vi "Main.vi"() -> ()   [LabVIEW 2021]
doc: "The myRIO Project template acquires acceleration data from the onboard accelerometer and displays the changes of acceleration values in a waveform chart."
panel:
  out "PLACEHOLDER\nLED control":dbl format="%#_13g"
  in  "PLACEHOLDER\nSfc Temp":dbl=150.0 format="%#_13g"
  out "Warmer\nON":bool
  out "HOT\nSurface":bool
  out "Surface Danger Level":string
  in  "Set-Temp-Slider":dbl(slide) scale=80.0..180.0
  out "Temp-Chart":T1(graph)
  in  "stop":bool
  # "Nice Warm Coffee"
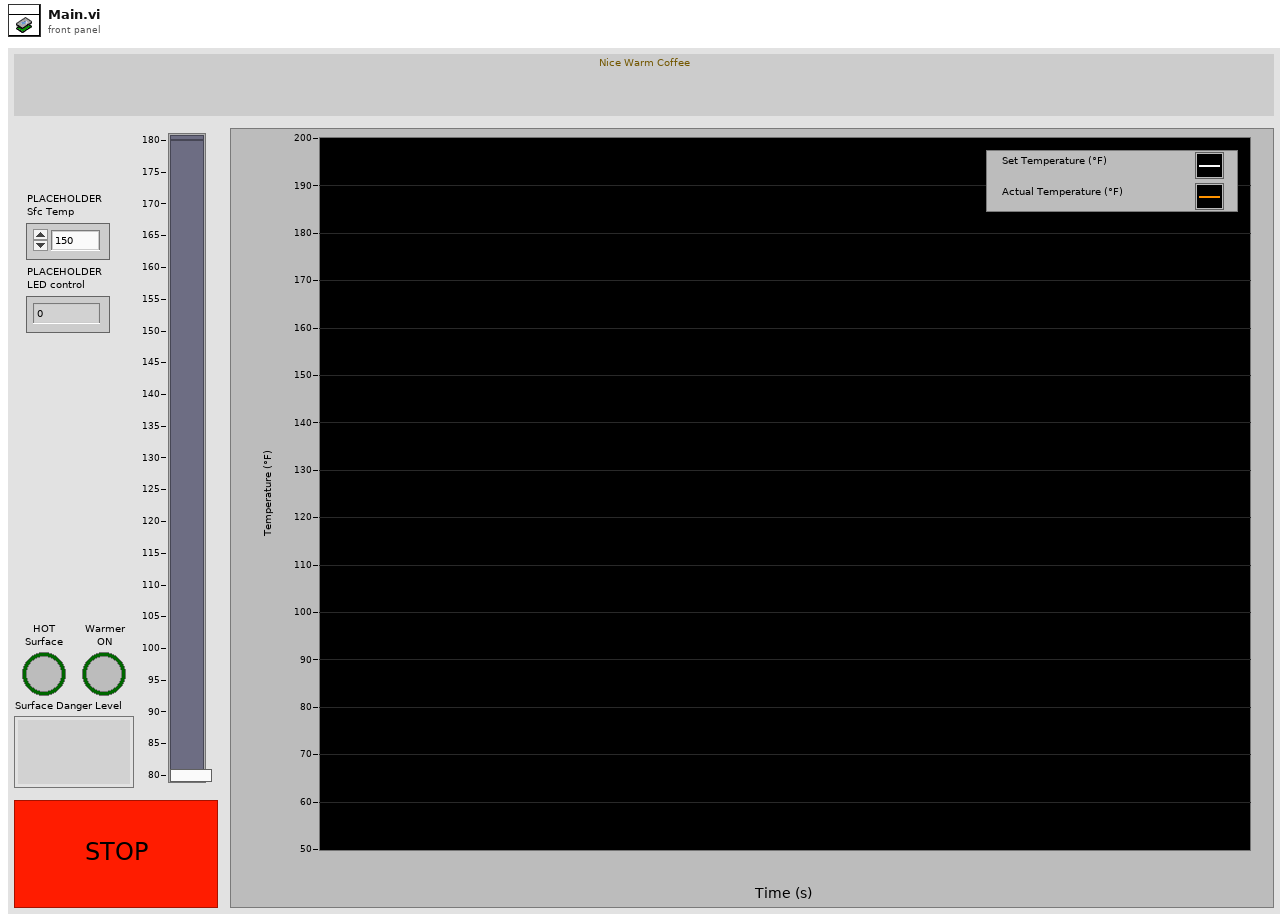
[diagram p1: front panel]
types:
  T1 = cluster{"[0]":dbl, "[1]":dbl, "[2]":dbl, "[3]":dbl, "[4]":dbl, "[5]":dbl, "[6]":dbl, "[7]":dbl, "[8]":dbl}
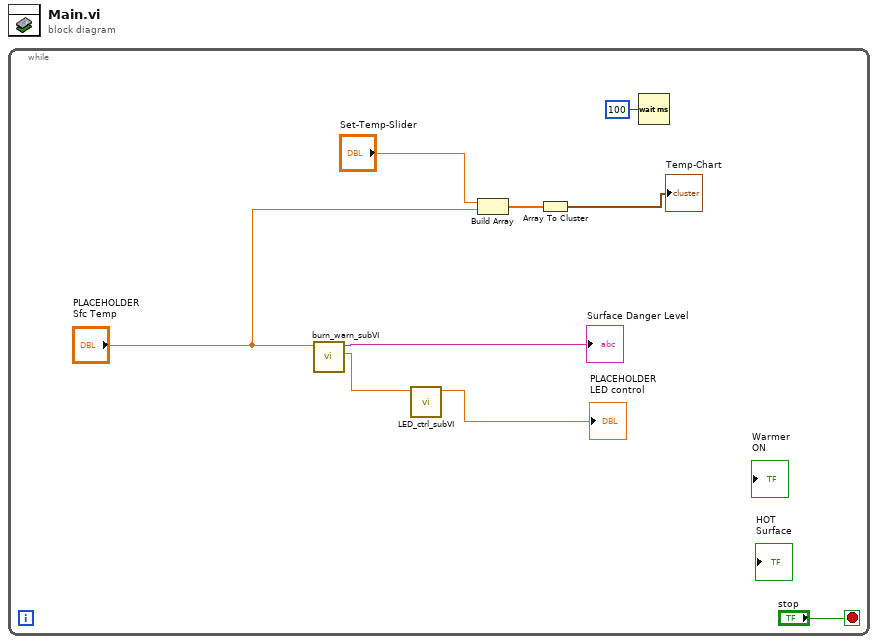
[diagram p0: block diagram]
diagram:
  n1 = while {
    stop <- "stop" stop-if-true
    n2 = call "burn_warn_subVI.vi"("Placeholder\nSfc Temp"="PLACEHOLDER\nSfc Temp") -> ("Numeric"=w2:dbl, "String"=→"Surface Danger Level":string)  [unwired: 9 in]
    n3 = call "LED_ctrl_subVI.vi"("Numeric in"=w2) -> ("Numeric out"=→"PLACEHOLDER\nLED control":dbl)  [unwired: 10 in]
    n4 = Build Array("Set-Temp-Slider", "PLACEHOLDER\nSfc Temp") -> (w5:dbl[])
    n5 = Array To Cluster(array=w5) -> (cluster=→"Temp-Chart":T1)
    n6 = Wait (ms)(milliseconds to wait=u32 100) -> ()  [unwired: 1 out]
  }
